vi "Update Connection Control by Reference.vi"(7 "Direction to Include":T1=enum."Publisher", 8 "error in (no error)":errorcluster, 10 "Channels":refnum<vi>, 11 "Channel Connection":refnum<vi>) -> (0 "error out":errorcluster, 2 "Channel Name":string)   [LabVIEW 2021, in "CIF_Manager_UI.lvclass"]
uses:
  CIF_Manager_UI.lvclass
  <vilib>/CIF Foundation/CIF Core/CIFUI/Typedef/Direction to Include.ctl
  Typedef/Channel Connection.ctl
  <vilib>/CIF Foundation/CIF Core/CIFCore/Common/CIFCoreCommon.lvlib
  <vilib>/CIF Foundation/CIF Core/CIFUI/CIF_UI.lvclass
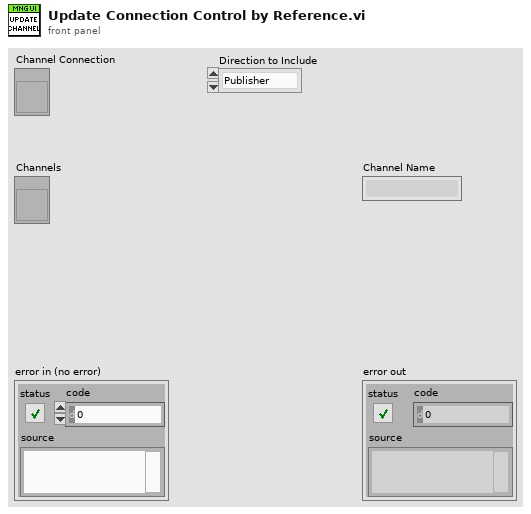
[diagram p1: front panel]
types:
  T1 = typedef "CIF_UI.lvclass/Direction to Include.ctl" = enum16{"All", "Subscriber", "Publisher"}
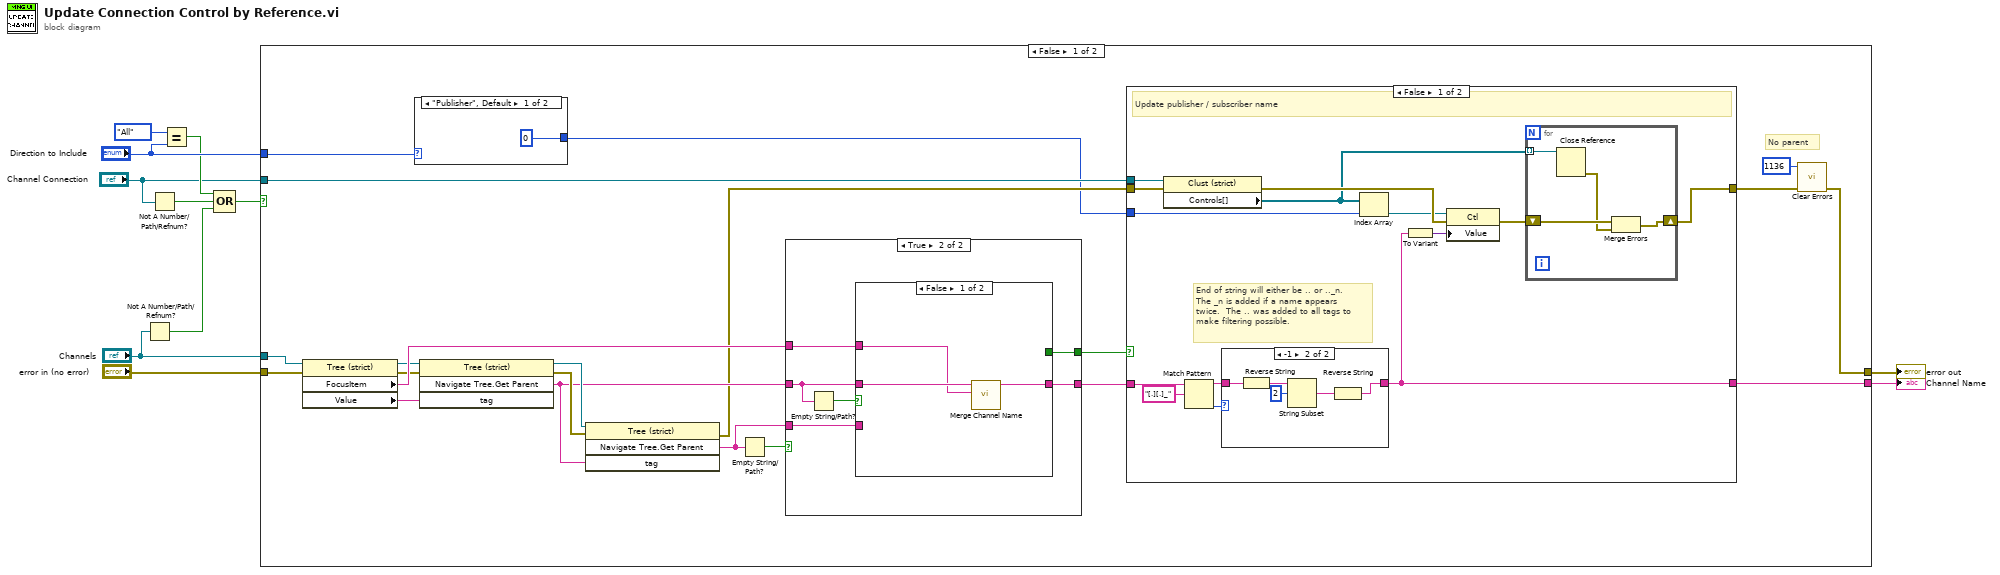
[diagram p0: block diagram]
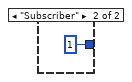
[diagram p2: hidden frame]
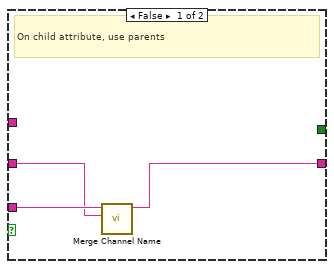
[diagram p5: hidden frame]
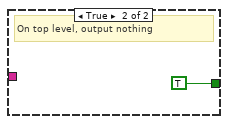
[diagram p6: hidden frame]
diagram:
  n1 = Not A Number/Path/Refnum?(number/path/refnum="Channels") -> (NaN/Path/Refnum?=w4:bool)
  n2 = Not A Number/Path/Refnum?(number/path/refnum="Channel Connection") -> (NaN/Path/Refnum?=w6:bool)
  n3 = Equal?(x=Direction_to_Include."All", y="Direction to Include") -> (x = y?=w5:bool)
  n4 = Compound Arithmetic op=OR(w5, w6, w4) -> (w3:bool)
  n5 = case shown="False" w3 {
    tunnel: "error in (no error)" -> [w26 w72]
    tunnel: [w18 w72] -> w10
    tunnel: "Channel Connection" -> [w16 _]
    tunnel: "Channels" -> [w15 _]
    tunnel: "Direction to Include" -> [w14 _]
    tunnel: [w12 _] -> w1
    frame False {
      # "No parent"
      n6 = property class="Tree (strict)"(reference=w15, error in=w26) -> (error out=w28:errorcluster, "FocusItem"=w29:string, "Value"=w31:string)  [unwired: 1 out]
      n7 = case shown="\"Publisher\", Default" w14 {
        tunnel: [0 ("index") 1 ("index")] -> w13
        frame "Publisher", Default {
        }
        frame "Subscriber" {
        }
      }
      n8 = invoke class="Tree (strict)" method="Navigate Tree.Get Parent"(reference=w15, error in=w28, "tag"=w31) -> (reference out=w25:refnum<vi>, error out=w24:errorcluster, "Navigate Tree:Get Parent"=w23:string)  [unwired: 1 in, 1 out]
      n9 = invoke class="Tree (strict)" method="Navigate Tree.Get Parent"(reference=w25, error in=w24, "tag"=w23) -> (error out=w20:errorcluster, "Navigate Tree:Get Parent"=w22:string)  [unwired: 1 in, 2 out]
      n10 = Empty String/Path?(string/path=w22) -> (empty?=w30:bool)
      n11 = case shown="True" w30 {
        tunnel: w23 -> [w59 w63]
        tunnel: w29 -> [_ w64]
        tunnel: [w61 w65] -> w27
        tunnel: w22 -> [w60 w62]
        tunnel: [_ w66] -> w21
        frame False {
          # "On child attribute, use parents"
          n12 = call <vilib>:"Merge Channel Name.vi"("Child"=w59, "Parent"=w60) -> ("Channel Name"=w61:string)  [unwired: 9 in]
        }
        frame True {
          n13 = Empty String/Path?(string/path=w63) -> (empty?=w67:bool)
          n14 = case shown="False" w67 {
            tunnel: [_ TRUE] -> w66
            tunnel: [w70 _] -> w65
            tunnel: w64 -> [w68 _]
            tunnel: w63 -> [w69 _]
            tunnel: w62 -> [_ _]
            frame False {
              n15 = call <vilib>:"Merge Channel Name.vi"("Child"=w68, "Parent"=w69) -> ("Channel Name"=w70:string)  [unwired: 9 in]
            }
            frame True {
              # "On top level, output nothing"
            }
          }
        }
      }
      n16 = case shown="False" w21 {
        tunnel: w27 -> [w41 _]
        tunnel: [w34 w58] -> w19
        tunnel: w16 -> [w46 _]
        tunnel: w20 -> [w43 w58]
        tunnel: w13 -> [w42 _]
        tunnel: [w37 _] -> w12
        frame False {
          # "End of string will either be .. or .._n.  The _n is added if a name appears twice.  The .. was added to all tags to make filtering possible."
          # "Update publisher / subscriber name"
          n17 = property class="Clust (strict)"(reference=w46, error in=w43) -> (error out=w47:errorcluster, "Controls[]"=w35:refnum<vi>[])  [unwired: 1 out]
          n18 = Match Pattern(string=w41, regular expression="[.][.]_") -> (before substring=w38:string, offset past match=w39:i32)  [unwired: 1 in, 2 out]
          n19 = case shown="-1" w39 {
            tunnel: w38 -> [w52 w57]
            tunnel: [w52 w53] -> w37
            frame 0, Default {
            }
            frame -1 {
              n20 = Reverse String(1:w57) -> (0:w56:string)
              n21 = String Subset(string=w56, offset (0)=2) -> (substring=w54:string)  [unwired: 1 in]
              n22 = Reverse String(1:w54) -> (0:w53:string)
            }
          }
          n23 = Index Array(array=w35, index=w42) -> (element=w44:refnum<vi>)
          n24 = To Variant(anything=w37) -> (Variant=w45:variant)
          n25 = property class="Ctl"(reference=w44, error in=w47, "Value"=w45) -> (error out=w36:errorcluster)  [unwired: 1 out]
          n26 = for {
            tunnel: w35 -> [w51] mode=indexing
            shift-right: [w48] -> w34
            shift-left: w36 -> [w50]
            n27 = Close Reference(reference=w51) -> (error out=w49:errorcluster)  [unwired: 1 in]
            n28 = Merge Errors(w50, w49) -> (w48:errorcluster)
          }
        }
        frame True {
        }
      }
      n29 = call <vilib>:"Clear Errors.vi"("error in (no error)"=w19, "specific error code to clear (0: all)"=1136) -> ("error out"=w18:errorcluster)  [unwired: 4 in, 1 out]
    }
    frame True {
    }
  }
  "error out" <- w10
  "Channel Name" <- w1
